vi "MB errors.vi"(10 "MB status":T3[](array[typedef]) {"MB update(s)" format="%.2g"; "ProCoDA Request"."PC update (s)" format="%.2f"; "ProCoDA Request"."# registers" min=1}, 11 "Devices":T2[](array[typedef])) -> (3 "MB errors":T1[](array[typedef]))   [LabVIEW 2019]
uses:
  MB status.ctl
  ProCoDA MB Request.ctl
  Read Write.ctl
  MB ID-Address.ctl
  MB error message.ctl
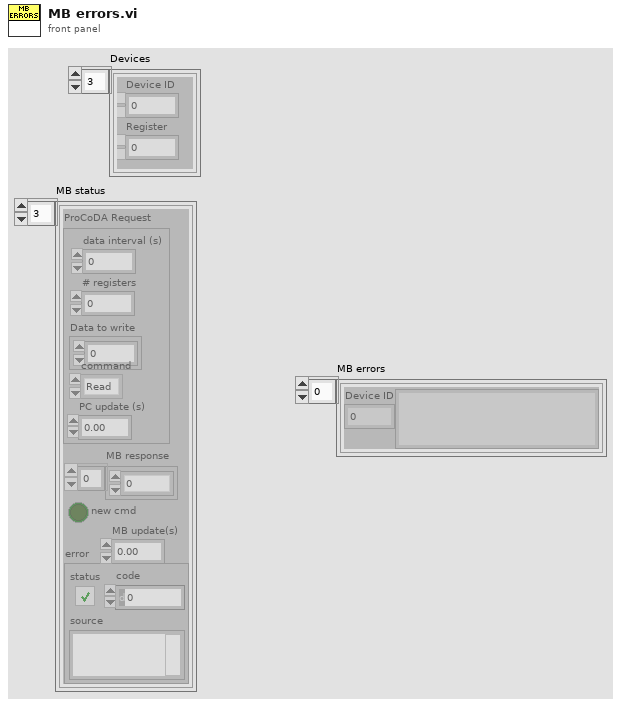
[diagram p1: front panel]
types:
  T1 = typedef "MB error message.ctl" = cluster{"message":string, "Device ID":u8}
  T2 = typedef "MB ID-Address.ctl" = cluster{"Device ID":u8, "Register":u16}
  T3 = typedef "MB status.ctl" = cluster{"ProCoDA Request":T4, "MB response":dbl[], "new cmd":bool, "error":errorcluster, "MB update(s)":dbl}
  T4 = typedef "ProCoDA MB Request.ctl" = cluster{"# registers":u8, "Data to write":u16[], "data interval (s)":dbl, "command":T5, "PC update (s)":dbl}
  T5 = typedef "Read Write.ctl" = enum16{"Read", "Write"}
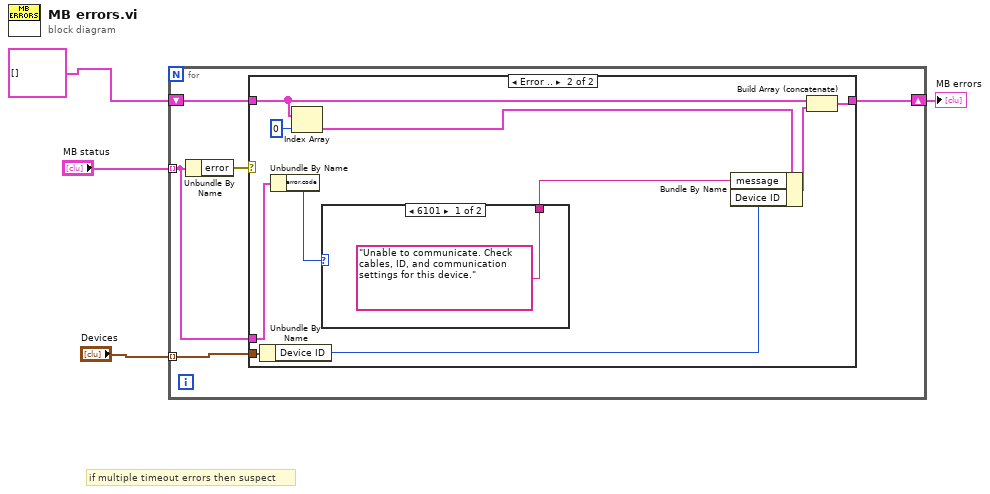
[diagram p0: block diagram]
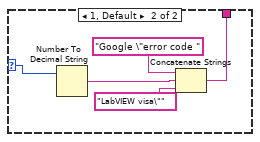
[diagram p3: hidden frame]
diagram:
  # "if multiple timeout errors then suspect"
  n1 = for {
    tunnel: "MB status" -> [w6] mode=indexing
    tunnel: "Devices" -> [w5] mode=indexing
    shift-right: [w7] -> w2
    shift-left: T1[] [] ("MB errors") -> [w9]
    n2 = Unbundle By Name(w6) -> ("error"=w8:errorcluster)
    n3 = case shown="Error .." w8 {
      tunnel: w9 -> [w10 w18]
      tunnel: [w10 w16] -> w7
      tunnel: w6 -> [_ w15]
      tunnel: w5 -> [_ w14]
      frame No Error {
      }
      frame Error {
        n4 = Unbundle By Name(w14) -> ("Device ID"=w13:u8)
        n5 = Unbundle By Name(w15) -> ("error.code"=w12:i32)
        n6 = Index Array(array=w18, index=0) -> (element=w19:T1)
        n7 = case shown="6101" w12 {
          selector: w12 -> [_ w26]
          tunnel: ["Unable to communicate. Check cables, ID, and communication settings for this device." w22] -> w11
          frame 6101 {
          }
          frame 1, Default {
            n8 = Number To Decimal String(number=w26) -> (decimal integer string=w24:string)  [unwired: 1 in]
            n9 = Concatenate Strings("Google \"error code ", w24, "LabVIEW visa\"" ("string")) -> (w22:string)
          }
        }
        n10 = Bundle By Name(cluster=w19, "message"=w11, "Device ID"=w13) -> (w17:T1)
        n11 = Build Array (concatenate)(w18, w17) -> (w16:T1[])
      }
    }
  }
  "MB errors" <- w2
